vi "LoRa.vi"(7 "LoRa Command":T2, 8 "error in (no error)":errorcluster, 9 "UART Connector":enum16{"UART0", "UART1"}(ring), 10 "Variant":variant, 11 "VISA resource name":refnum<visa-resource-name>="COM15") -> (0 "error out":errorcluster, 1 "read buffer":string, 2 "Returned Data":string[](array[string]), 3 "VISA resource name out":refnum<visa-resource-name>, 4 "Identity":T1)   [LabVIEW 2024]
uses:
  LoRaCommands.ctl
  Parameter.ctl
  Bandwidth.ctl
  Payload.ctl
  Band.ctl
  Baudrates.ctl
  Message.ctl
  2544c41a-67d0-46c8-811c-b9ee5a9b367d.vi
  10365c10-e032-4fe0-ada6-100d9b40629b.vi
  <vilib>/Utility/error.llb/Trim Whitespace One-Sided.vi
  Driver/CTIPicoVISA.lvlib
panel:
  # "Input"
  # "Output"
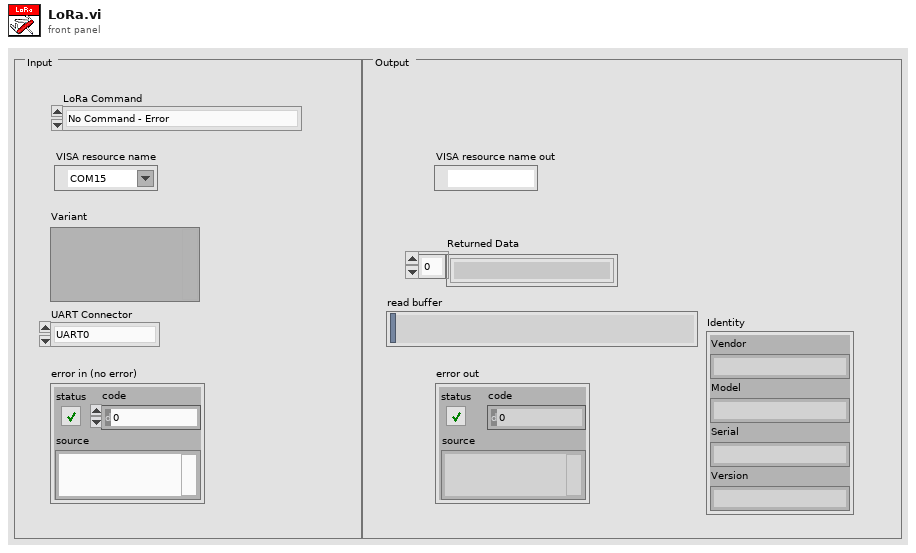
[diagram p1: front panel]
types:
  T1 = cluster{"Vendor":string, "Model":string, "Serial":string, "Version":string}
  T2 = typedef "LoRaCommands.ctl" = enum16{"No Command - Error", "Connect", "check radio present(AT)", "Software Reset", "Set Work Mode TXRX(AT+MODE=0)", "Set Work Mode Sleep(AT+MODE=1)", "Get Work Mode(AT+MODE?)", "Set UART Baudrate", "Get UART Baudrate", "Set RF Frequency", "Get RF Frequency", "Set Module Address(AT+ADDRESS=<Addr>)", "Get Module Address(AT+ADDRESS?)", "Set Network ID(AT+NETWORKID=<ID>)", "Get Network ID(AT+NETWORKID?)", "Set Network PWD(AT+CPIN=<PW>)", "Get Network PWD(AT+CPIN?)", "Set RF OP Power(AT+CRFOP=<power>)", "Get RF OP Power(AT+CRFOP?)", "Send Data", "Receive Data", "Get Firmware Version", "Get UID of Module(AT+UID?)", "Set To Factory Defaults(AT+FACTORY)", "Set Spreading Factor", "Get Spreading Factor", "Set Bandwidth", "Get Bandwidth", "Set Coding Rate", "Get Coding Rate", "Set Preamble", "Get Preamble", "Set Active Region", "Get Active Region", "Get RF Parameters", "Set RF Parameters", "Write Message", "Disconnect"}
  T3 = typedef "Parameter.ctl" = cluster{"Bandwidth":T4, "Spreading Factor (7-12)":u8, "Coding Rate (1-4)":u8, "Programmed Preamble(4-7)":u8}
  T4 = typedef "Bandwidth.ctl" = enum16{"125kHz", "250kHz", "500kHz", "7.8kHz", "10.4kHz", "15.6kHz", "20.8kHz", "31.25kHz", "41.7kHz", "62.5kHz"}
  T5 = typedef "Payload.ctl" = cluster{"Address":i32, "Data":string}
  T6 = typedef "Baudrates.ctl" = enum16{"300", "1200", "4800", "9600", "19200", "28800", "38400", "57600", "115200"}
  T7 = typedef "Message.ctl" = cluster{"Message":string, "Expected Response":string}
  T8 = typedef "Band.ctl" = enum16{"EU433", "CN470", "RU864", "IN865", "EU868", "US915", "AU915", "KR920", "AS923-1", "AS923-2", "AS923-3", "AS923-4", "LA915"}
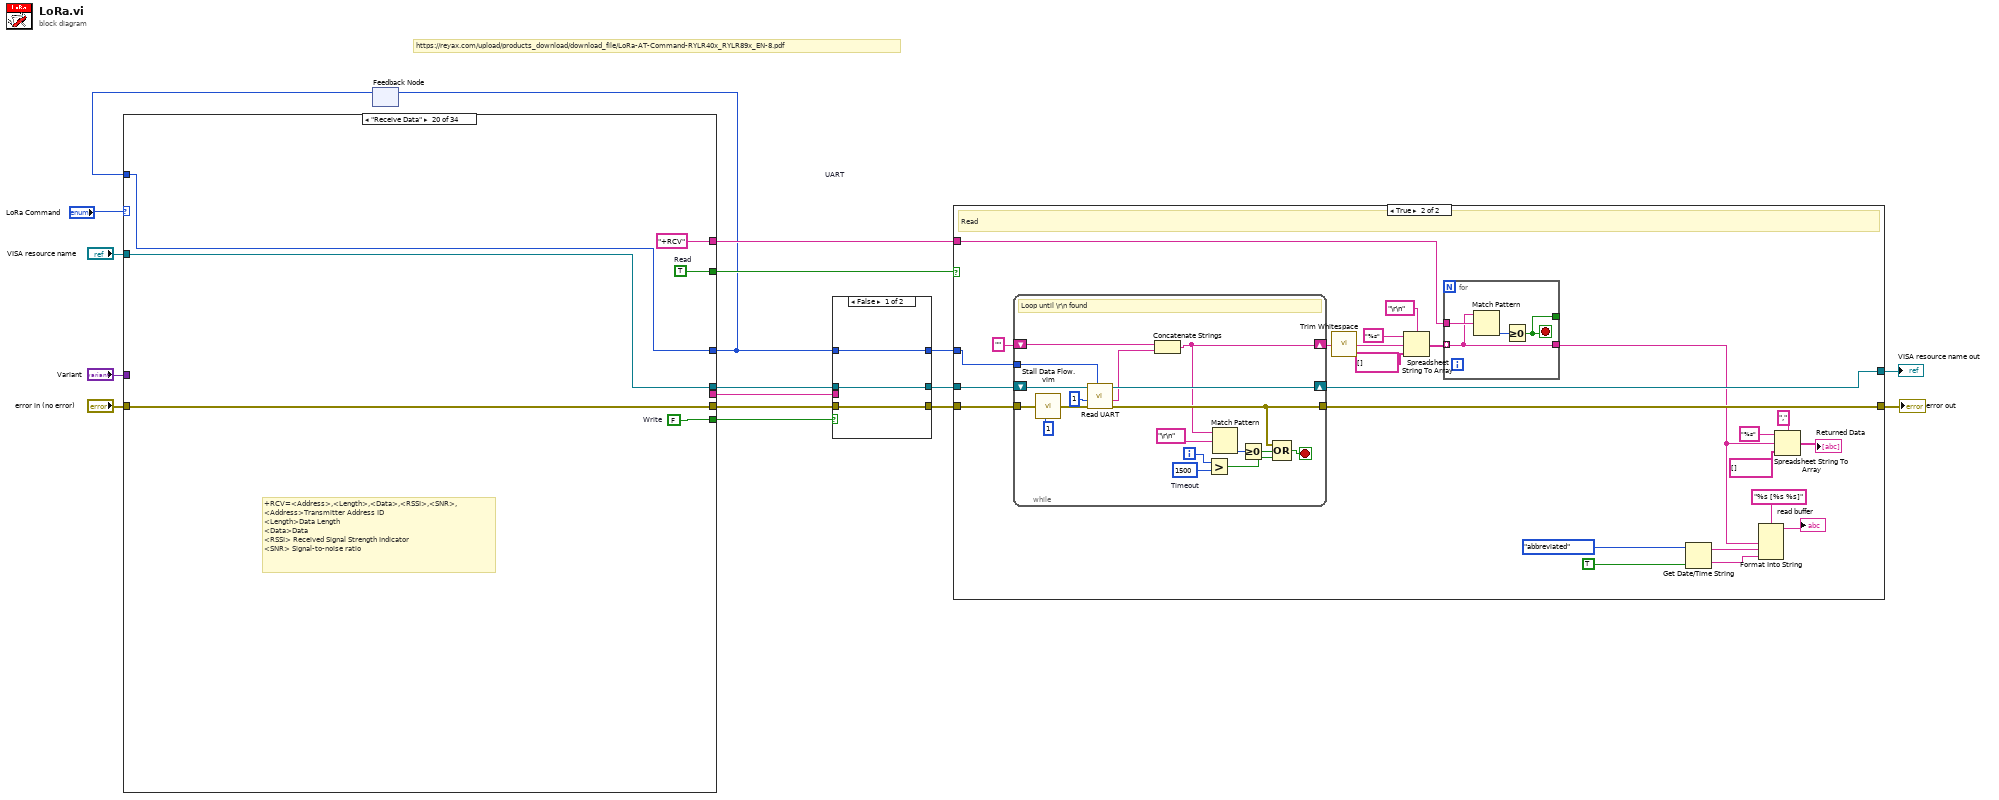
[diagram p0: block diagram]
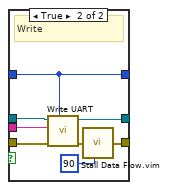
[diagram p3: hidden frame]
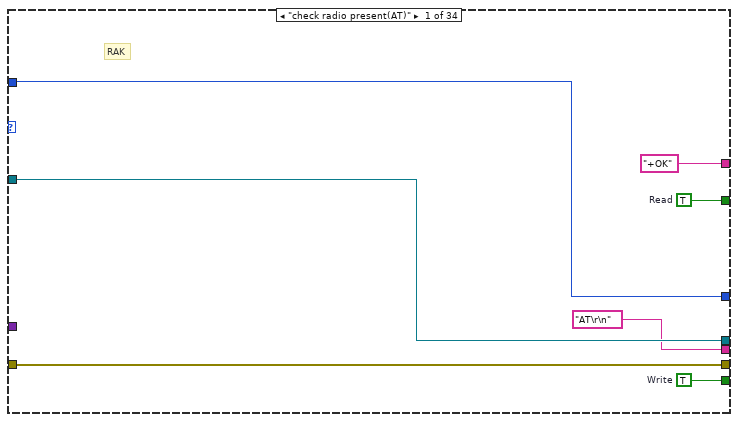
[diagram p4: hidden frame]
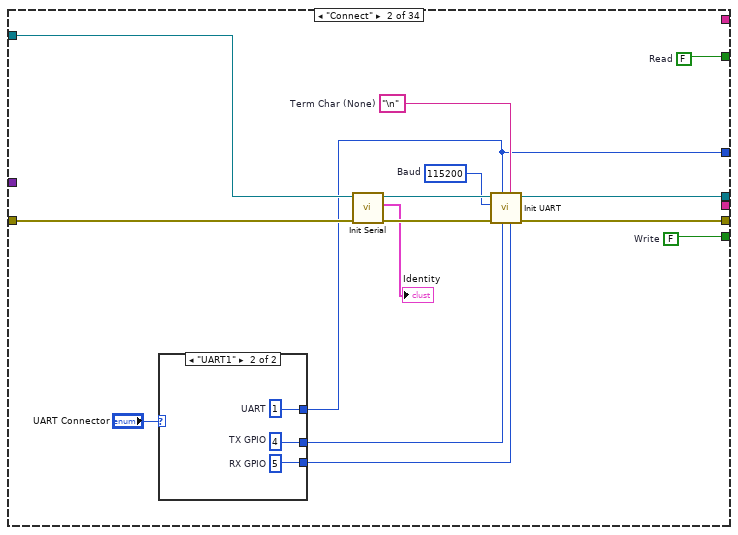
[diagram p5: hidden frame]
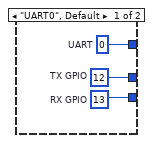
[diagram p6: hidden frame]
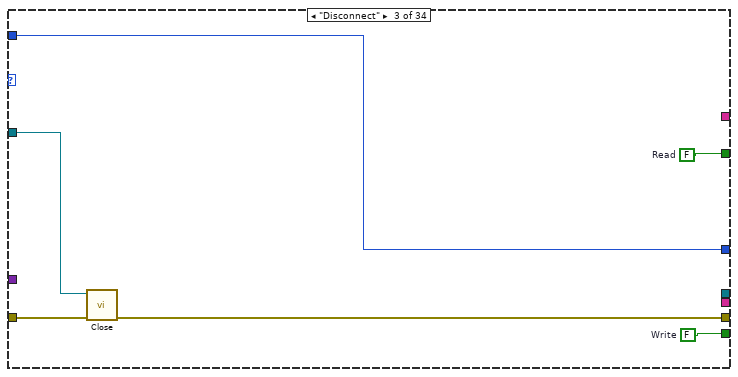
[diagram p7: hidden frame]
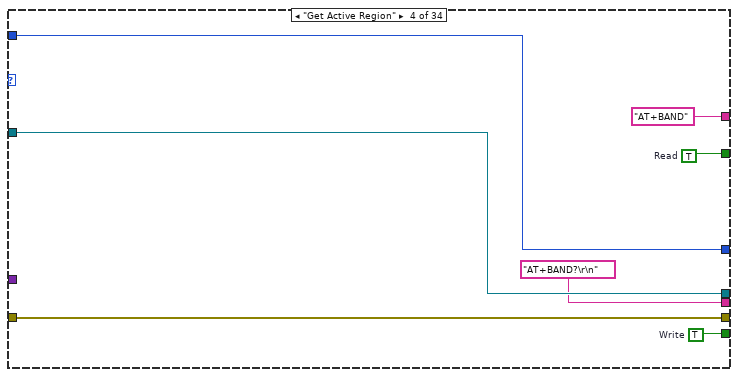
[diagram p8: hidden frame]
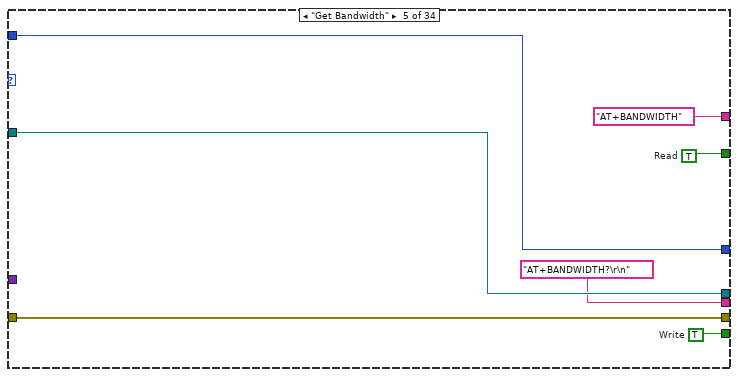
[diagram p9: hidden frame]
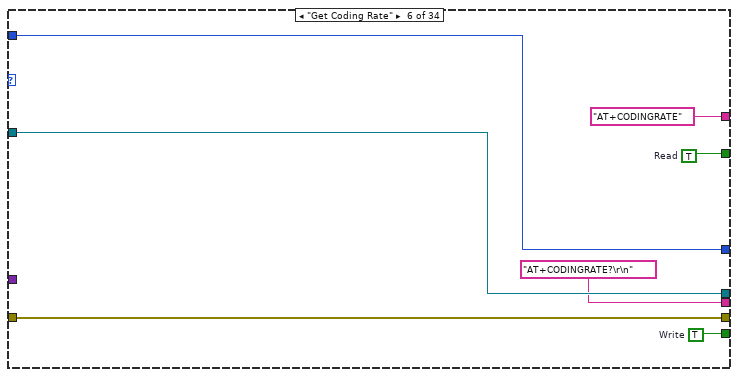
[diagram p10: hidden frame]
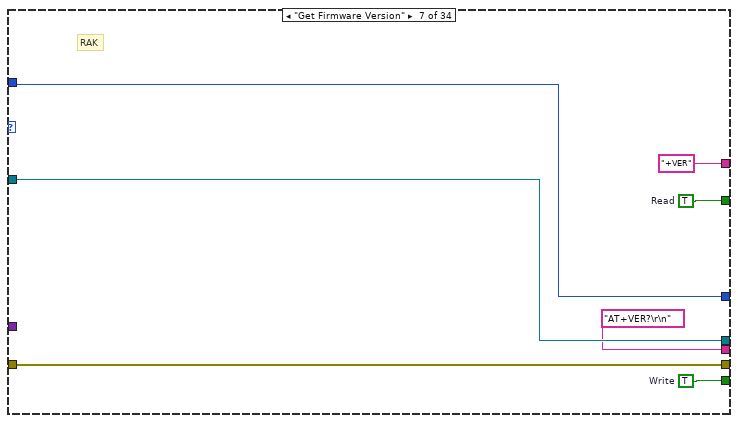
[diagram p11: hidden frame]
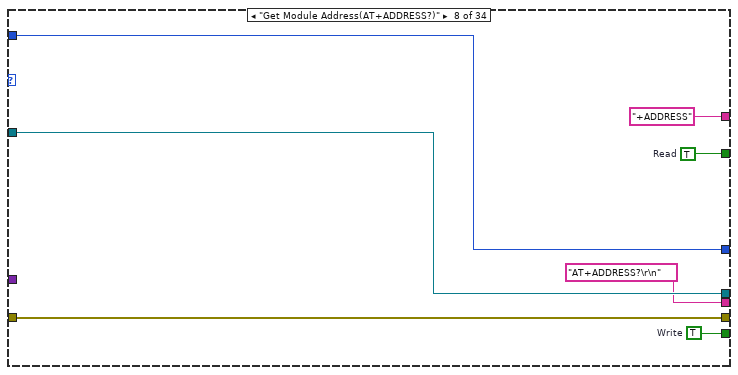
[diagram p12: hidden frame]
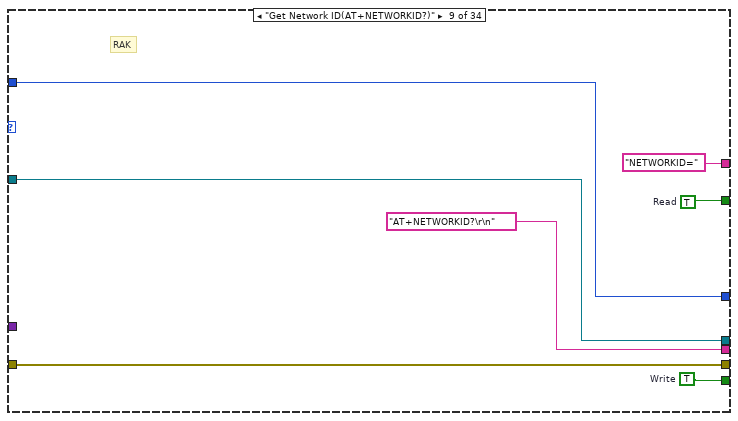
[diagram p13: hidden frame]
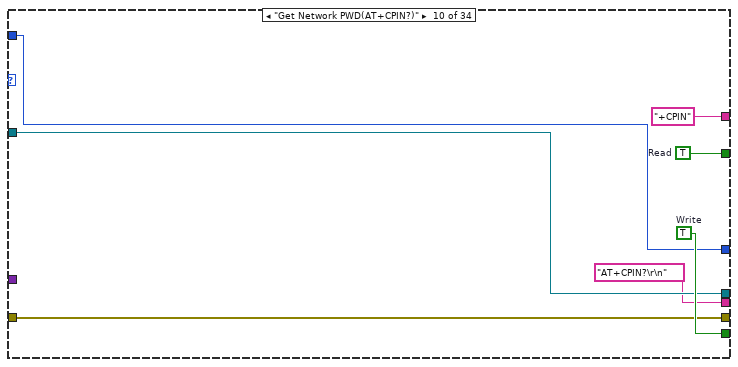
[diagram p14: hidden frame]
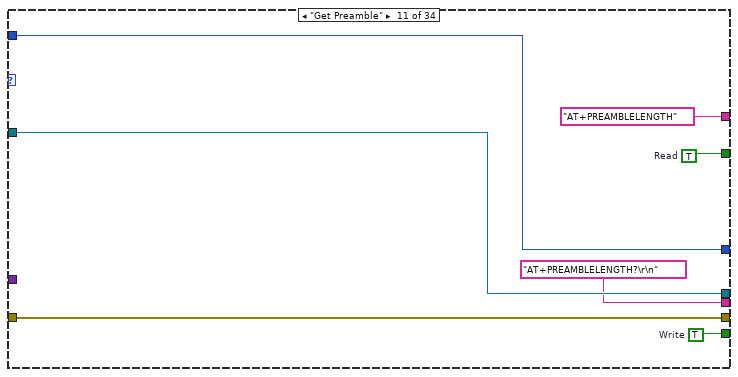
[diagram p15: hidden frame]
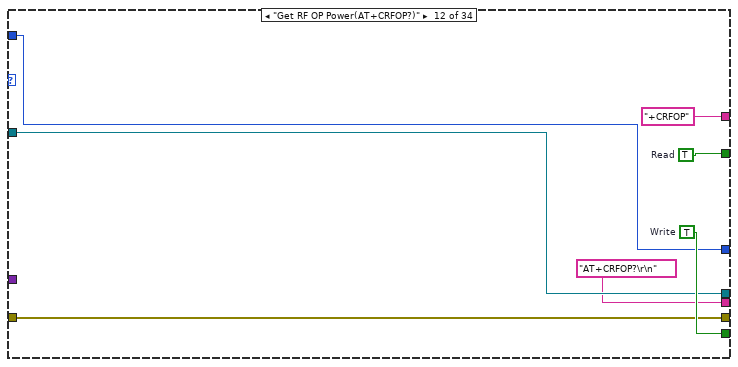
[diagram p16: hidden frame]
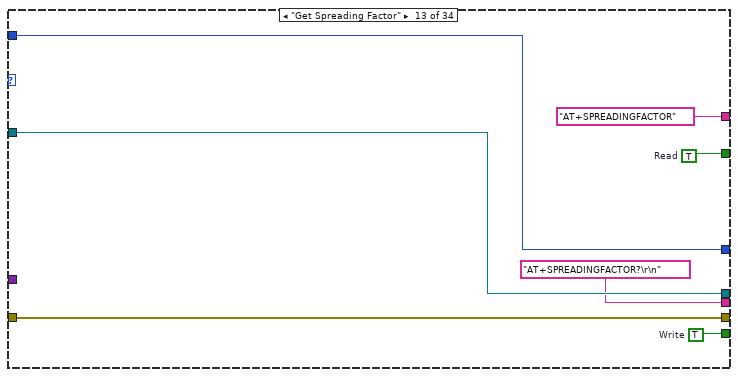
[diagram p17: hidden frame]
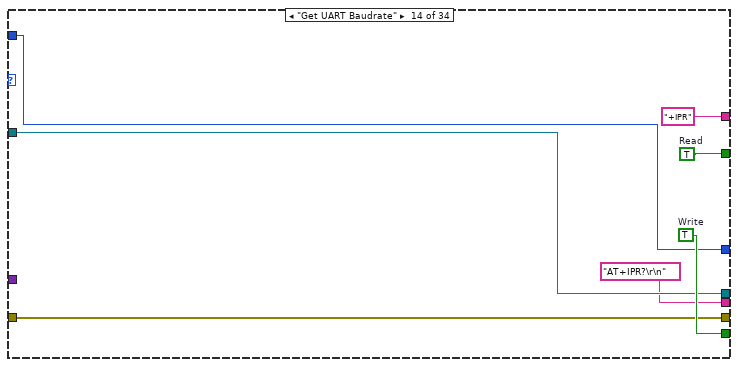
[diagram p18: hidden frame]
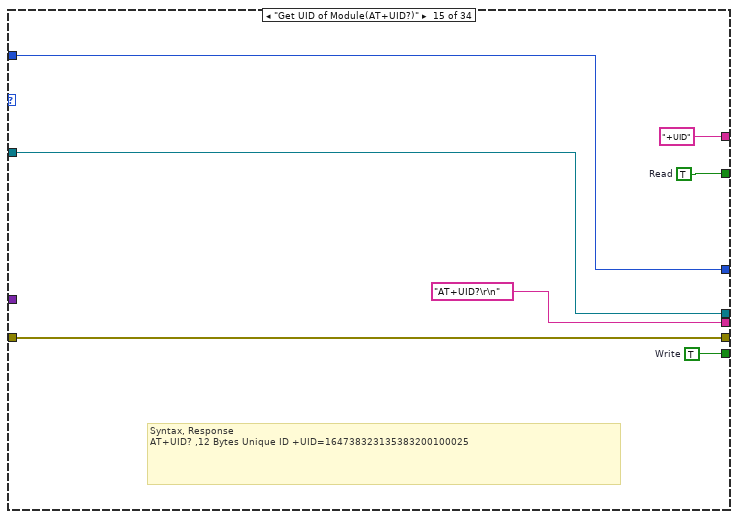
[diagram p19: hidden frame]
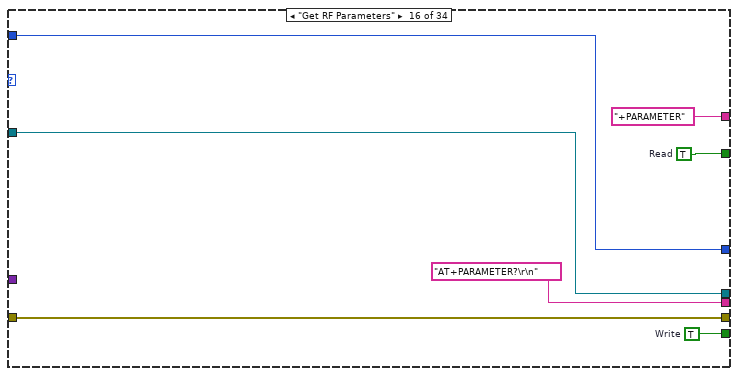
[diagram p20: hidden frame]
diagram:
  # "https://reyax.com/upload/products_download/download_file/LoRa-AT-Command-RYLR40x_RYLR89x_EN-8.pdf"
  n1 = feedback #1 "UART"() -> (w1:u8)  [unwired: 1 in]
  n2 = case shown="\"Receive Data\"" "LoRa Command" {
    tunnel: "Variant" -> [_ _ _ _ _ _ _ _ _ _ _ _ _ _ _ _ w146 _ _ _ w187 w199 w211 w224 w237 w246 w260 w272 _ w293 _ _ _ w326]
    tunnel: "error in (no error)" -> [w22 w32 w48 w56 w63 w70 w77 w84 w91 w98 w105 w112 w119 w126 w133 w140 w147 w163 w169 w174 w188 w200 w212 w225 w238 w245 w261 w273 w282 w294 w303 w310 w317 w327]
    tunnel: [w22 w30 w47 w56 w63 w70 w77 w84 w91 w98 w105 w112 w119 w126 w133 w140 w145 w163 w169 w174 w186 w198 w210 w223 w236 w244 w259 w271 w282 w292 w303 w310 w317 w325] -> w11
    tunnel: [w21 w29 _ w55 w62 w69 w76 w83 w90 w97 w104 w111 w118 w125 w132 w139 w156 w162 w170 w173 w189 w202 w215 w227 w239 w251 w263 w275 w281 w296 w302 w309 w316 w328] -> w10
    tunnel: "VISA resource name" -> [w21 w31 w49 w55 w62 w69 w76 w83 w90 w97 w104 w111 w118 w125 w132 w139 w156 w162 w170 w173 w189 w202 w215 w227 w239 w251 w263 w275 w281 w296 w302 w309 w316 w328]
    tunnel: [w23 w38 w50 w57 w64 w71 w78 w85 w92 w99 w106 w113 w120 w127 w134 w141 w157 w164 w168 w175 w190 w203 w216 w228 w240 w252 w264 w276 w283 w297 w304 w311 w318 w329] -> w7
    tunnel: [w24 w39 w51 w58 w65 w72 w79 w86 w93 w100 w107 w114 w121 w128 w135 w142 w158 w165 w167 w176 w191 w204 w217 w229 w241 w253 w265 w277 w284 w298 w305 w312 w319 w330] -> w6
    tunnel: ["AT\r\n" _ _ "AT+BAND?\r\n" "AT+BANDWIDTH?\r\n" "AT+CODINGRATE?\r\n" "AT+VER?\r\n" "AT+ADDRESS?\r\n" "AT+NETWORKID?\r\n" "AT+CPIN?\r\n" "AT+PREAMBLELENGTH?\r\n" "AT+CRFOP?\r\n" "AT+SPREADINGFACTOR?\r\n" "AT+IPR?\r\n" "AT+UID?\r\n" "AT+PARAMETER?\r\n" w148 "AT+MODE?\r\n" _ _ w177 w197 w213 w222 w231 w242 w258 w270 "AT+ATR\r\n" w291 "AT+SLEEP\r\n" "AT+MODE=0\r\n" "AT+ATZ\r\n" w321] -> w5
    tunnel: ["+OK" _ _ "AT+BAND" "AT+BANDWIDTH" "AT+CODINGRATE" "+VER" "+ADDRESS" "NETWORKID=" "+CPIN" "AT+PREAMBLELENGTH" "+CRFOP" "AT+SPREADINGFACTOR" "+IPR" "+UID" "+PARAMETER" "+OK" "+" _ "+RCV" "+OK" "AT+BAND" "OK" "+OK" "+OK" "+OK" "+OK" "+OK" "OK" "OK" "OK" "+OK" "OK" w320] -> w4
    tunnel: [w18 w27 w46 w52 w59 w66 w73 w80 w87 w94 w101 w108 w115 w122 w129 w136 w154 w159 w166 w171 w182 w194 w208 w218 w233 w249 w254 w266 w278 w285 w299 w306 w313 w324] -> w2
    tunnel: w1 -> [w18 _ w46 w52 w59 w66 w73 w80 w87 w94 w101 w108 w115 w122 w129 w136 w154 w159 w166 w171 w182 w194 w208 w218 w233 w249 w254 w266 w278 w285 w299 w306 w313 w324]
    frame "check radio present(AT)" {
      w24 = TRUE  # Read
      w23 = TRUE  # Write
      # "RAK"
    }
    frame "Connect" {
      w34 = "\n"  # Term Char (None)
      w35 = u32 115200  # Baud
      w39 = FALSE  # Read
      w38 = FALSE  # Write
      n3 = case shown="\"UART1\"" "UART Connector" {
        tunnel: [w42 w43] -> w26
        tunnel: [w41 w44] -> w25
        tunnel: [w40 w45] -> w27
        frame "UART0", Default {
          w41 = u8 13  # RX GPIO
          w42 = u8 12  # TX GPIO
          w40 = u8 0  # UART
        }
        frame "UART1" {
          w44 = u8 5  # RX GPIO
          w43 = u8 4  # TX GPIO
          w45 = u8 1  # UART
        }
      }
      n4 = call "Init Serial.vi"("error in (no error)"=w32, "VISA resource name in"=w31) -> ("error out"=w36:errorcluster, "Identity"=→"Identity":T1, "VISA resource name Out"=w37:refnum<visa-resource-name>)  [unwired: 7 in]
      n5 = call "Init UART.vi"("RX GPIO"=w25, "Term Char (None)"=w34, "TX GPIO"=w26, "UART"=w27, "error in (no error)"=w36, "Baud"=w35, "VISA resource name in"=w37) -> ("error out"=w30:errorcluster, "VISA resource name"=w29:refnum<visa-resource-name>)  [unwired: 3 in]
    }
    frame "Disconnect" {
      w51 = FALSE  # Read
      w50 = FALSE  # Write
      n6 = call "Close.vi"("error in (no error)"=w48, "VISA resource name in"=w49) -> ("error out"=w47:errorcluster)  [unwired: 9 in]
    }
    frame "Get Active Region" {
      w58 = TRUE  # Read
      w57 = TRUE  # Write
    }
    frame "Get Bandwidth" {
      w65 = TRUE  # Read
      w64 = TRUE  # Write
    }
    frame "Get Coding Rate" {
      w72 = TRUE  # Read
      w71 = TRUE  # Write
    }
    frame "Get Firmware Version" {
      w79 = TRUE  # Read
      w78 = TRUE  # Write
      # "RAK"
    }
    frame "Get Module Address(AT+ADDRESS?)" {
      w86 = TRUE  # Read
      w85 = TRUE  # Write
    }
    frame "Get Network ID(AT+NETWORKID?)" {
      w93 = TRUE  # Read
      w92 = TRUE  # Write
      # "RAK"
    }
    frame "Get Network PWD(AT+CPIN?)" {
      w100 = TRUE  # Read
      w99 = TRUE  # Write
    }
    frame "Get Preamble" {
      w107 = TRUE  # Read
      w106 = TRUE  # Write
    }
    frame "Get RF OP Power(AT+CRFOP?)" {
      w114 = TRUE  # Read
      w113 = TRUE  # Write
    }
    frame "Get Spreading Factor" {
      w121 = TRUE  # Read
      w120 = TRUE  # Write
    }
    frame "Get UART Baudrate" {
      w128 = TRUE  # Read
      w127 = TRUE  # Write
    }
    frame "Get UID of Module(AT+UID?)" {
      w135 = TRUE  # Read
      w134 = TRUE  # Write
      # "Syntax, Response\nAT+UID? ,12 Bytes Unique ID +UID=164738323135383200100025"
    }
    frame "Get RF Parameters" {
      w142 = TRUE  # Read
      w141 = TRUE  # Write
    }
    frame "Set RF Parameters" {
      w158 = TRUE  # Read
      w157 = TRUE  # Write
      # "AT+PARAMETER=<Spreading Factor>,\n<Bandwidth>,<Coding Rate>,\n<Programmed Preamble>\n<Spreading Factor>7~12, (default 12)\n<Bandwidth>0~9 list as below\n0 : 7.8KHz (not recommended, over spec.)\n1 : 10.4KHz (not recommended, over spec.)\n2 : 15.6KHz\n3 : 20.8 KHz\n4 : 31.25 KHz\n5 : 41.7 KHz\n6 : 62.5 KHz\n7 : 125 KHz (default).\n8 : 250 KHz\n9 : 500 KHz\n<Coding Rat>1~4, (default 1)\n<Programmed Preamble> 4~7(default 4)\nExample : Set the parameters as below:\n<Spreading Factor> 7,<Bandwidth> 20.8KHz,\n<Coding Rate> 4,<Programmed Preamble>5,\nAT+PARAMETER=7,3,4,5"
      n7 = Variant To Data(error in=w147, type=T3 {"Bandwidth"=enum."7.8kHz", "Spreading Factor (7-12)"=12, "Coding Rate (1-4)"=1, "Programmed Preamble(4-7)"=4} ("Parameter"), Variant=w146) -> (data=w143:T3, error out=w145:errorcluster)
      n8 = Unbundle By Name(w143) -> ("Spreading Factor (7-12)"=w150:u8, "Bandwidth"=w151:T4, "Coding Rate (1-4)"=w152:u8, "Programmed Preamble(4-7)"=w153:u8)
      n9 = Format Into String(format string="AT+PARAMETER=%d,%d,%d,%d\r\n", w150, w151, w152, w153) -> (resulting string=w148:string)  [unwired: 2 in, 1 out]
    }
    frame "Get Work Mode(AT+MODE?)" {
      w165 = TRUE  # Read
      w164 = TRUE  # Write
      # "#TODO need to check 2 options here, which is a bit clunky"
      # "AT+MODE?\nAny text\n+MODE=0 for Transmit and Receive mode\n+READY for Sleep mode"
    }
    frame "No Command - Error", Default {
      w167 = FALSE  # Read
      w168 = FALSE  # Write
    }
    frame "Receive Data" {
      w176 = TRUE  # Read
      w175 = FALSE  # Write
      # "+RCV=<Address>,<Length>,<Data>,<RSSI>,<SNR>,\n<Address>Transmitter Address ID\n<Length>Data Length\n<Data>Data\n<RSSI> Received Signal Strength Indicator\n<SNR> Signal-to-noise ratio"
    }
    frame "Send Data" {
      w191 = TRUE  # Read
      w190 = TRUE  # Write
      # "AT+SEND=<Address>,<Payload Length>,<Data>\n<Address>0~65535, When the <Address> is 0,\nit will send data to all address (From 0 to 65535.)\n<Payload Length>Maximum 240bytes\n<Data>ASCII Format\nExample : Send HELLO string to the Address 50,\nAT+SEND=50,5,HELLO"
      n10 = Variant To Data(error in=w188, type=T5 {"Address"=0, "Data"=""} ("Payload"), Variant=w187) -> (data=w184:T5, error out=w186:errorcluster)
      n11 = Unbundle By Name(w184) -> ("Address"=w179:i32, "Data"=w178:string)
      n12 = String Length(string=w178) -> (length=w180:i32)
      n13 = Format Into String(format string="AT+SEND=%d,%d,%s\r\n", w179, w180, w178) -> (resulting string=w177:string)  [unwired: 2 in, 1 out]
    }
    frame "Set Active Region" {
      w193 = Band."AS923-1"  # Band
      w204 = TRUE  # Read
      w203 = TRUE  # Write
      # "RAK"
      n14 = Variant To Data(error in=w200, type=w193, Variant=w199) -> (data=w196:T8, error out=w198:errorcluster)
      n15 = To Unsigned Byte Integer(number=w196) -> (unsigned 8bit integer=w192:u8)
      n16 = Format Into String(format string="AT+BAND=%d\r\n", w192) -> (resulting string=w197:string)  [unwired: 2 in, 1 out]
    }
    frame "Set Bandwidth" {
      w207 = Bandwidth."7.8kHz"  # Bandwidth
      w217 = TRUE  # Read
      w216 = TRUE  # Write
      n17 = Variant To Data(error in=w212, type=w207, Variant=w211) -> (data=w206:T4, error out=w210:errorcluster)
      n18 = To Unsigned Byte Integer(number=w206) -> (unsigned 8bit integer=w205:u8)
      n19 = Format Into String(format string="AT+BANDWIDTH%d\r\n", w205) -> (resulting string=w213:string)  [unwired: 2 in, 1 out]
    }
    frame "Set Module Address(AT+ADDRESS=<Addr>)" {
      w221 = 1  # Address
      w229 = TRUE  # Read
      w228 = TRUE  # Write
      # "AT+ADDRESS=<Address>\n<Address>=0~65535(default 0)\nExample : Set the address of module as 120,\n*The settings will be memorized in EEPROM.\nAT+ADDRESS=120"
      n20 = Variant To Data(error in=w225, type=w221, Variant=w224) -> (data=w220:i32, error out=w223:errorcluster)
      n21 = Format Into String(format string="AT+ADDRESS=%d\r\n", w220) -> (resulting string=w222:string)  [unwired: 2 in, 1 out]
    }
    frame "Set Network ID(AT+NETWORKID=<ID>)" {
      w235 = 1  # NetworkID
      w241 = TRUE  # Read
      w240 = TRUE  # Write
      # "AT+NETWORKID=<Network ID>\n<Network ID>0~16(default 0)\nExample : Set the network ID as 6,\n*The settings will be memorized in EEPROM.\n*The”0”is the public ID of Lora. It is not\nrecommend to set 0 to make the distinction of\nNETWORK.\nAT+NETWORKID=6"
      n22 = Variant To Data(error in=w238, type=w235, Variant=w237) -> (data=w230:i32, error out=w236:errorcluster)
      n23 = Format Into String(format string="AT+NETWORKID=%d\r\n", w230) -> (resulting string=w231:string)  [unwired: 2 in, 1 out]
    }
    frame "Set RF Frequency" {
      w248 = 868500000  # Frequency
      w253 = TRUE  # Read
      w252 = TRUE  # Write
      # "AT+BAND=<parameter>\n<parameter>is the RF Frequency, Unit is Hz\n470000000: 470000000Hz(default: RYLR40x)\n915000000: 915000000Hz(default: RYLY89x)\nExample : Set the frequency as 868500000Hz,\nAT+BAND=868500000"
      n24 = Variant To Data(error in=w245, type=w248, Variant=w246) -> (data=w247:i32, error out=w244:errorcluster)
      n25 = Format Into String(format string="AT+BAND=%d\r\n", w247) -> (resulting string=w242:string)  [unwired: 2 in, 1 out]
    }
    frame "Set Network PWD(AT+CPIN=<PW>)" {
      w257 = ""  # PWD
      w265 = TRUE  # Read
      w264 = TRUE  # Write
      # "AT+CPIN=<Password>\n<Password>: An 32 character long AES password\nFrom 00000000000000000000000000000001 to\nFFFFFFFFFFFFFFFFFFFFFFFFFFFFFFFF\nOnly by using same password can the data be\nrecognized.\nAfter resetting, the previously password will\ndisappear.\nExample : Set the password as below:\nFABC0002EEDCAA90FABC0002EEDCAA90\nAT+CPIN=FABC0002EEDCAA90FABC0002EEDCAA90"
      n26 = Variant To Data(error in=w261, type=w257, Variant=w260) -> (data=w256:string, error out=w259:errorcluster)
      n27 = Format Into String(format string="AT+CPIN=%s\r\n", w256) -> (resulting string=w258:string)  [unwired: 2 in, 1 out]
    }
    frame "Set RF OP Power(AT+CRFOP=<power>)" {
      w269 = 1  # POWER
      w277 = TRUE  # Read
      w276 = TRUE  # Write
      # "AT+CRFOP=<power>\n<power>0~15\n15:15dBm(default)\n14:14dBm\n……\n01:1dBm\n00:0dBm\nExample: Set the output power as 10dBm,\nAT+CRFOP=10"
      n28 = Variant To Data(error in=w273, type=w269, Variant=w272) -> (data=w268:i32, error out=w271:errorcluster)
      n29 = Format Into String(format string="AT+CRFOP=%d\r\n", w268) -> (resulting string=w270:string)  [unwired: 2 in, 1 out]
    }
    frame "Set To Factory Defaults(AT+FACTORY)" {
      w284 = TRUE  # Read
      w283 = TRUE  # Write
      # "RAK"
    }
    frame "Set UART Baudrate" {
      w298 = TRUE  # Read
      w297 = TRUE  # Write
      # "AT+IPR=<rate>\n<rate> is the UART baud rate:\n300\n1200\n4800\n9600\n19200\n28800\n38400\n57600\n115200(default).\nExample: Set the baud rate as 9600,\n*The settings will be memorized in EEPROM.\nAT+IPR=9600"
      n30 = Variant To Data(error in=w294, type=Baudrates."115200", Variant=w293) -> (data=w288:T6, error out=w292:errorcluster)
      n31 = Index Array(array=i32[] [300, 1200, 4800, 9600, 19200, 28800, 38400, 57600, 115200], index=w288) -> (element=w287:i32)
      n32 = Format Into String(format string="AT+IPR=%d\r\n", w287) -> (resulting string=w291:string)  [unwired: 2 in, 1 out]
    }
    frame "Set Work Mode Sleep(AT+MODE=1)" {
      w305 = TRUE  # Read
      w304 = TRUE  # Write
      # "RAK"
    }
    frame "Set Work Mode TXRX(AT+MODE=0)" {
      w312 = TRUE  # Read
      w311 = TRUE  # Write
      # "#TODO HOW DO WE WAKE IT UP AGAIN"
    }
    frame "Software Reset" {
      w319 = TRUE  # Read
      w318 = TRUE  # Write
      # "RAK"
      # "Software Reset ? is this the same as load default"
      # "#TODO confirm what this does"
    }
    frame "Write Message" {
      w330 = TRUE  # Read
      w329 = TRUE  # Write
      # "AT+ADDRESS=<Address>\n<Address>=0~65535(default 0)\nExample : Set the address of module as 120,\n*The settings will be memorized in EEPROM.\nAT+ADDRESS=120"
      n33 = Variant To Data(error in=w327, type=T7 {"Message"="", "Expected Response"=""} ("Message"), Variant=w326) -> (data=w322:T7, error out=w325:errorcluster)
      n34 = Unbundle By Name(w322) -> ("Expected Response"=w320:string, "Message"=w321:string)
    }
  }
  n35 = feedback-in #1(w2) -> ()
  n36 = case shown="False" w7 {
    tunnel: [w332 w335] -> w14
    tunnel: [w333 w338] -> w13
    tunnel: w11 -> [w332 w339]
    tunnel: w10 -> [w333 w341]
    tunnel: w5 -> [_ w340]
    tunnel: w2 -> [w331 w336]
    tunnel: [w331 w336] -> w3
    frame False {
    }
    frame True {
      # "Write"
      n37 = call "Write UART.vi"("UART"=w336, "error in (no error)"=w339, "Data"=w340, "VISA resource name in"=w341) -> ("error out"=w337:errorcluster, "VISA resource name"=w338:refnum<visa-resource-name>)  [unwired: 6 in]
      n38 = call "Stall Data Flow.vim"("value in"=w337, "milliseconds to wait"=u32 90) -> ("value out"=w335:errorcluster)  [unwired: 1 out]
    }
  }
  n39 = case shown="True" w6 {
    tunnel: w14 -> [w342 w367]
    tunnel: w13 -> [w343 w366]
    tunnel: [w342 w359] -> w12
    tunnel: [w343 w358] -> w9
    tunnel: w4 -> [_ w352]
    tunnel: w3 -> [_ w353]
    frame False {
    }
    frame True {
      # "Read"
      n40 = while {
        shift-right: [w381] -> w358
        shift-left: w366 -> [w378]
        shift-right: [w372] -> w350
        shift-left: "" -> [w389]
        tunnel: w367 -> [w375]
        tunnel: [w380] -> w359
        tunnel: w353 -> [w377]
        i -> [w384]
        stop <- w386 stop-if-true
        w383 = 1500  # Timeout
        # "Loop until \\r\\n found"
        n41 = call "Stall Data Flow.vim"("value in"=w375, "milliseconds to wait"=u32 1) -> ("value out"=w374:errorcluster)  [unwired: 1 out]
        n42 = call "Read UART.vi"("UART"=w377, "error in (no error)"=w374, "Len (LineTerm)"=u8 1, "VISA resource name in"=w378) -> ("error out"=w380:errorcluster, "Data"=w379:string, "VISA resource name"=w381:refnum<visa-resource-name>)  [unwired: 5 in]
        n43 = Concatenate Strings(w389, w379) -> (w372:string)
        n44 = Greater?(x=w384, y=w383) -> (0:w382:bool)
        n45 = Match Pattern(string=w372, regular expression="\r\n") -> (offset past match=w388:i32)  [unwired: 1 in, 3 out]
        n46 = Greater Or Equal To 0?(x=w388) -> (x >= 0?=w387:bool)
        n47 = Compound Arithmetic op=OR(w380, w387, w382) -> (w386:bool)
      }
      n48 = call <vilib>:"Trim Whitespace.vi"("string"=w350) -> ("trimmed string"=w344:string)  [unwired: 1 in]
      n49 = Spreadsheet String To Array(delimiter (Tab)="\r\n", format string="%s", spreadsheet string=w344, array type (2D Dbl)=string[] []) -> (array=w345:string[])
      n50 = for {
        tunnel: w345 -> [w370] mode=indexing
        tunnel: w352 -> [w371]
        tunnel: [w370] -> w351
        tunnel: [w368] -> _
        stop <- w368 stop-if-true
        n51 = Match Pattern(string=w370, regular expression=w371) -> (offset past match=w369:i32)  [unwired: 1 in, 3 out]
        n52 = Greater Or Equal To 0?(x=w369) -> (x >= 0?=w368:bool)
      }
      n53 = Get Date/Time String(date format (0)=enum16{"short", "long", "abbreviated"}."abbreviated", want seconds? (F)=TRUE) -> (date string=w363:string, time string=w362:string)  [unwired: 1 in]
      n54 = Format Into String(format string="%s [%s %s]", w351, w363, w362) -> (resulting string=→"read buffer":string)  [unwired: 2 in, 1 out]
      n55 = Spreadsheet String To Array(delimiter (Tab)=",", format string="%s", spreadsheet string=w351, array type (2D Dbl)=string[] []) -> (array=→"Returned Data":string[])
    }
  }
  "error out" <- w12
  "VISA resource name out" <- w9
